vi "EndCheck Scan Code.vi"(8 "error in (no error)":errorcluster, 11 "Main":T1={"Tite"="", "Base path"=path "", "Table"=[], "Stations"=[], "Shield Array"=[], "UPHs"=[], "VISA"={"VISA"="", "baud rate"=9600, "data bits"=8, "parity"=enum."None", "stop bits"=10, "flow control"=0}, "Path"={"roof"=path "", "Config"=path "", "Png"=path ""}, "Ctr"={"DB Dispaly"=refnum, "Error Table"=refnum, "Display"=refnum, "Login"=refnum, "Exit"=refnum, "FTT_Submit"=refnum}, "Login"={"User"="", "Grade"=""}, "information"={"cause"="", "Type"=enum."Inform", "code"=0, "Suroce"="", "Status"=FALSE}, "Local DB"={"Connstr"="", "Database"={"Constr"={"Driver"="", "Server"="", "User"="", "Pwd"="", "Database"=""}, "conn ref"=refnum, "State"=FALSE}}, "Remote DB"={"Connstr"="", "Database"={"Constr"={"Driver"="", "Server"="", "User"="", "Pwd"="", "Database"=""}, "conn ref"=refnum, "State"=FALSE}}, "FTT TV"="", "ExchangeTime"=0, "NVH"="", "EOL Path"=path ""} {"VISA"."flow control" items=["None", "XON/XOFF", "RTS/CTS", "XON/XOFF & RTS/CTS", "DTR/DSR", "XON/XOFF & DTR/DSR"]; "VISA"."stop bits" items=["1.0"=10, "1.5"=15, "2.0"=20]}) -> (0 "error out":errorcluster)   [LabVIEW 2014]
uses:
  Type'def/Online_Table.ctl
  <vilib>/Instr/_visa.llb/VISA Flush IO Buffer Mask.ctl
  <vilib>/addons/database/_DB Variant To Data/Database Variant To Data.xnode
  Type'def/FTT Display Type.ctl
  Type'def/UPH Config.ctl
  VISA/Ctr/VISA Ctr.ctl
  Type'def/Main Ctr Ref.ctl
  Type'def/User Login.ctl
  Database/Ctr/Constr.ctl
  <vilib>/addons/database/Connection.llb/Conn ObjectReference.ctl
  <vilib>/addons/database/NI_Database_API.lvlib
  Database/Ctr/Conneect State.ctl
  Type'def/MainCtr.ctl
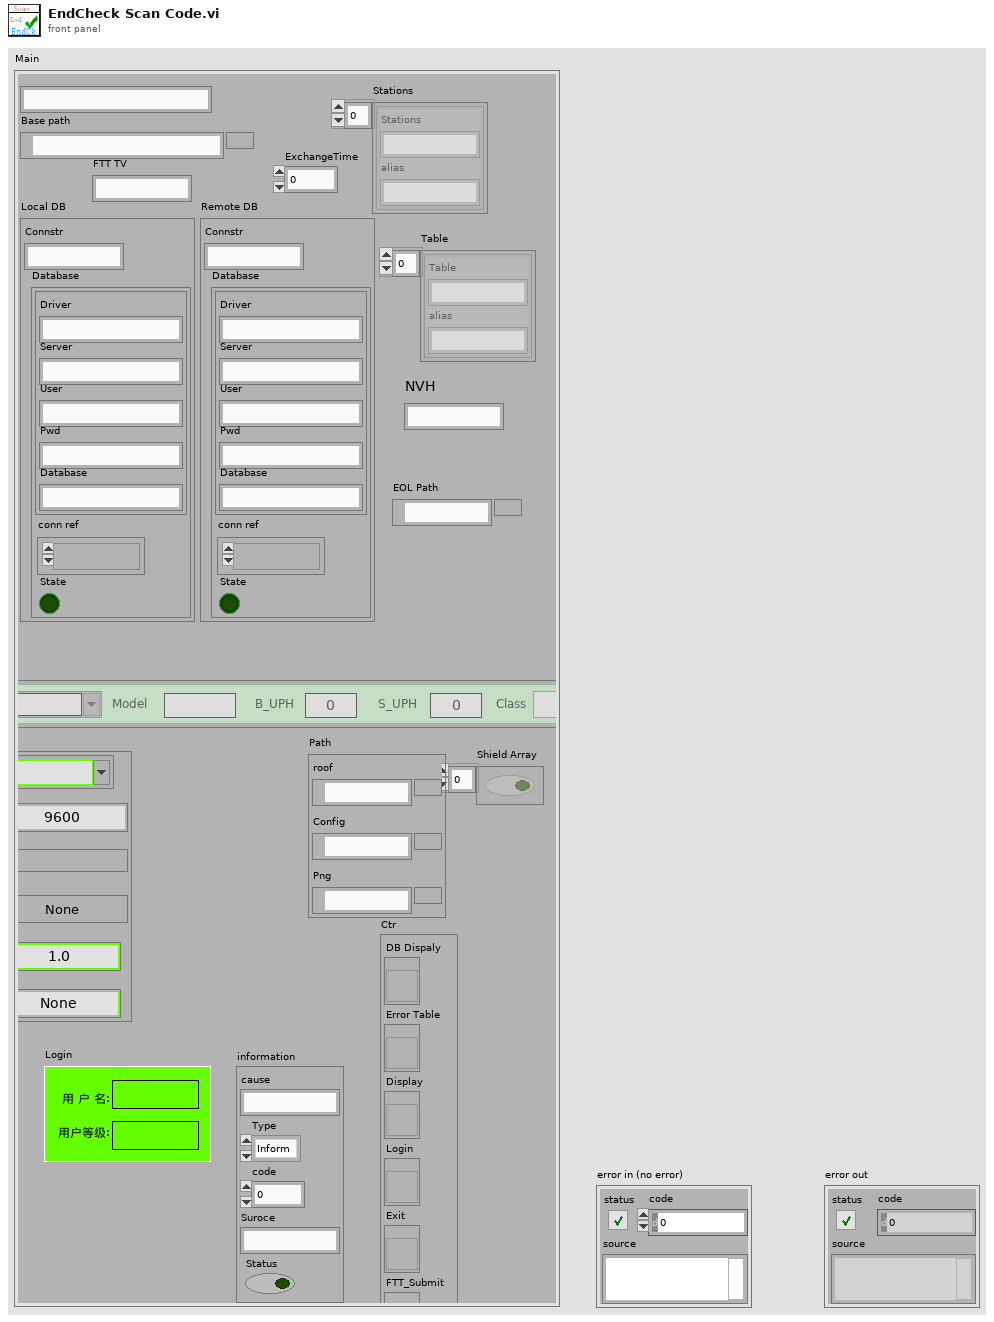
[diagram p1: front panel]
types:
  T1 = typedef "MainCtr.ctl" = cluster{"Tite":string, "Base path":path, "Table":cluster{"Table":string, "alias":string}[], "Stations":cluster{"Stations":string, "alias":string}[], "Shield Array":bool[], "UPHs":T2[], "VISA":T3, "Path":cluster{"roof":path, "Config":path, "Png":path}, "Ctr":T4, "Login":T5, "information":cluster{"cause":string, "Type":enum16{"Inform", "Warning", "Alarm"}, "code":i32, "Suroce":string, "Status":bool}, "Local DB":cluster{"Connstr":string, "Database":T6}, "Remote DB":cluster{"Connstr":string, "Database":T6}, "FTT TV":string, "ExchangeTime":i32, "NVH":string, "EOL Path":path}
  T2 = typedef "UPH Config.ctl" = cluster{"Line_No":string, "Model":string, "B_UPH ":i16, "S_UPH  ":i16, "Class":enum16{"Big", "Small"}}
  T3 = typedef "VISA Ctr.ctl" = cluster{"VISA":refnum<visa-resource-name>, "baud rate":u32, "data bits":u16, "parity":enum16{"None", "Odd", "Even", "Mark", "Space"}, "stop bits":u16, "flow control":u16}
  T4 = typedef "Main Ctr Ref.ctl" = cluster{"DB Dispaly":refnum<vi>, "Error Table":refnum<vi>, "Display":refnum<vi>, "Login":refnum<vi>, "Exit":refnum<vi>, "FTT_Submit":refnum<vi>}
  T5 = typedef "User Login.ctl" = cluster{"User":string, "Grade":string}
  T6 = typedef "Conneect State.ctl" = cluster{"Constr":T7, "conn ref":T8, "State":bool}
  T7 = typedef "Constr.ctl" = cluster{"Driver":string, "Server":string, "User":string, "Pwd":string, "Database":string}
  T8 = typedef "NI_Database_API.lvlib/Conn ObjectReference.ctl" = refnum<k1>
  T9 = typedef "FTT Display Type.ctl" = cluster{"Line.No":string, "Model":string, "Color":string, "UPH":dbl, "Plan":dbl, "Target Rate":dbl, "Target ":dbl, "Actual":dbl, "FTT":dbl, "FTT Rate":dbl, "Repaired":dbl, "Reject":dbl, "Ouline":dbl, "Line State":string}
  T10 = cluster{"cause":string, "Type":enum16{"Inform", "Warning", "Alarm"}, "code":i32, "Suroce":string, "Status":bool}
  T11 = typedef "Online_Table.ctl" = cluster{"SN":string, "Frame":string, "Station":string, "Model":string, "Color":string, "OnTime":timestamp, "OutTime":timestamp, "Repaired":i32, "OnRepair":bool, "Pstate":string}
  T12 = cluster{"Display":T9, "Main ":T1, "Online_Table":T11, "information":cluster{"cause":string, "Type":enum16{"Inform", "Warning", "Alarm"}, "code":i32, "Suroce":string, "Status":bool}}
  T13 = typedef "VISA Flush IO Buffer Mask.ctl" = u16
  T14 = cluster{"Display":T9, "Class":enum16{"Big", "Small"}}
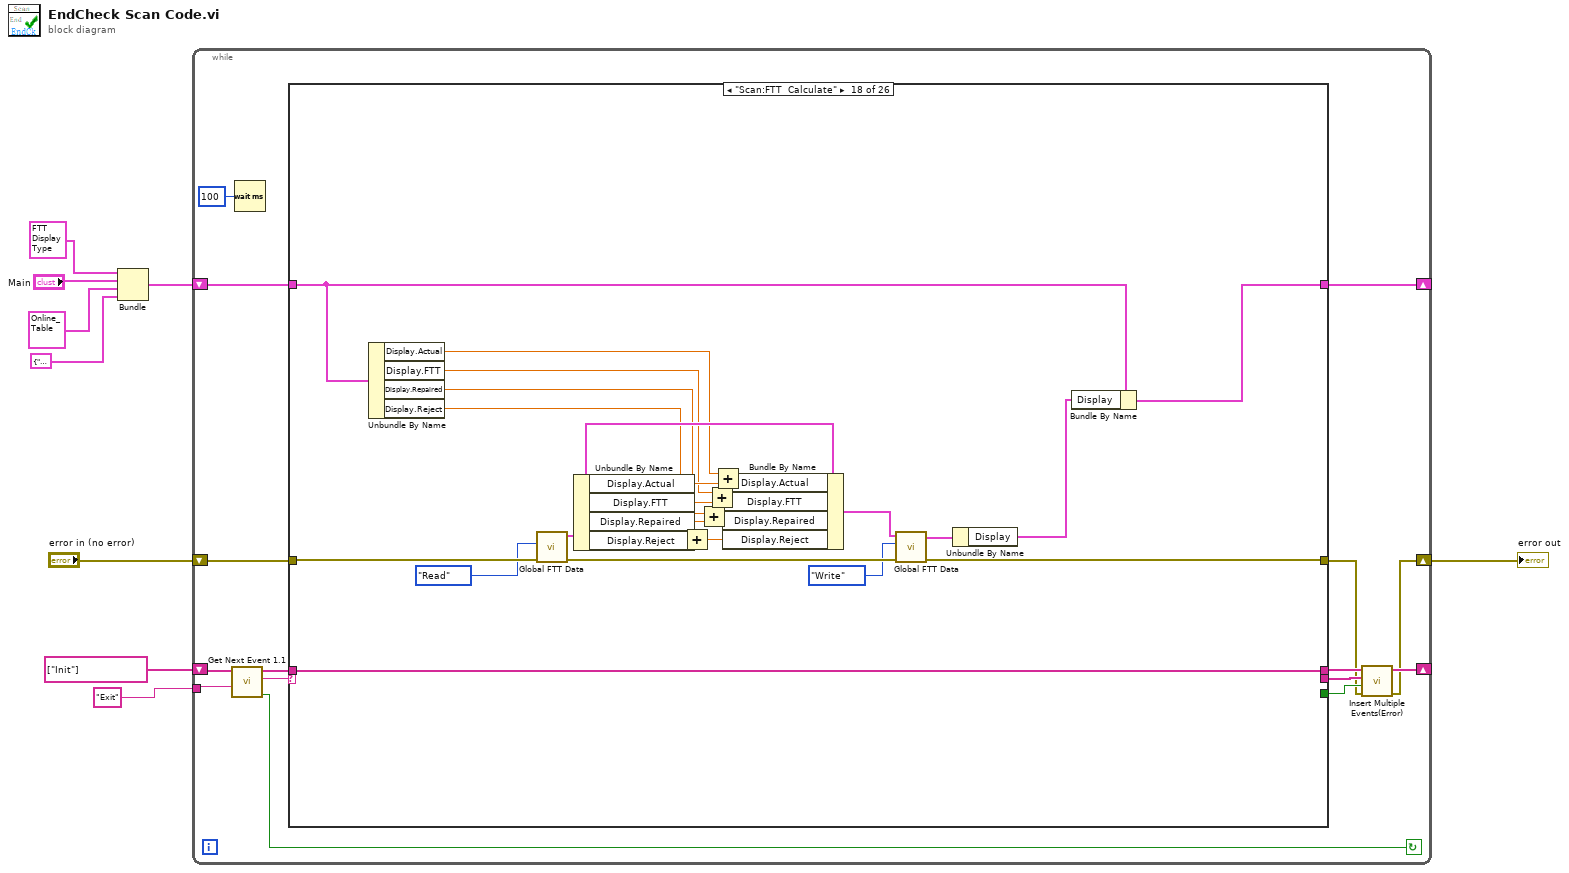
[diagram p0: block diagram]
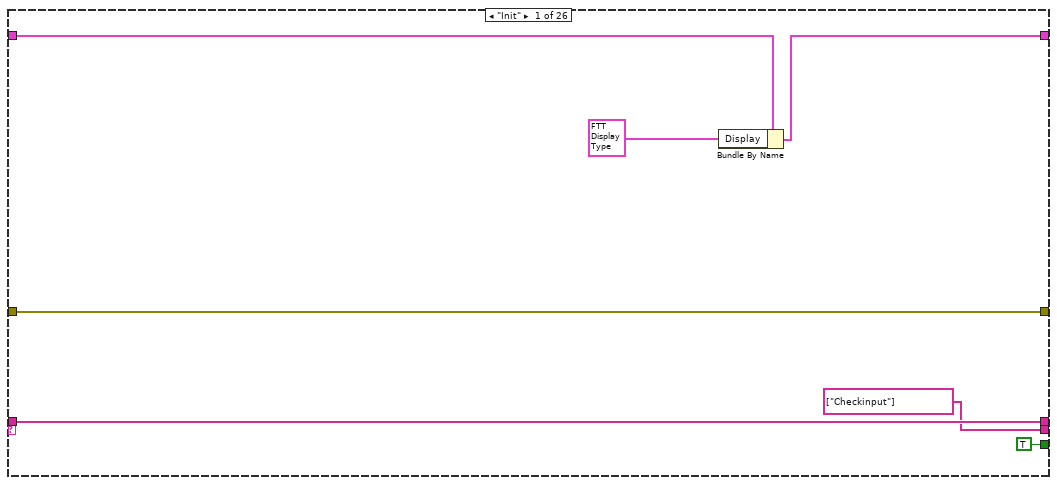
[diagram p2: hidden frame]
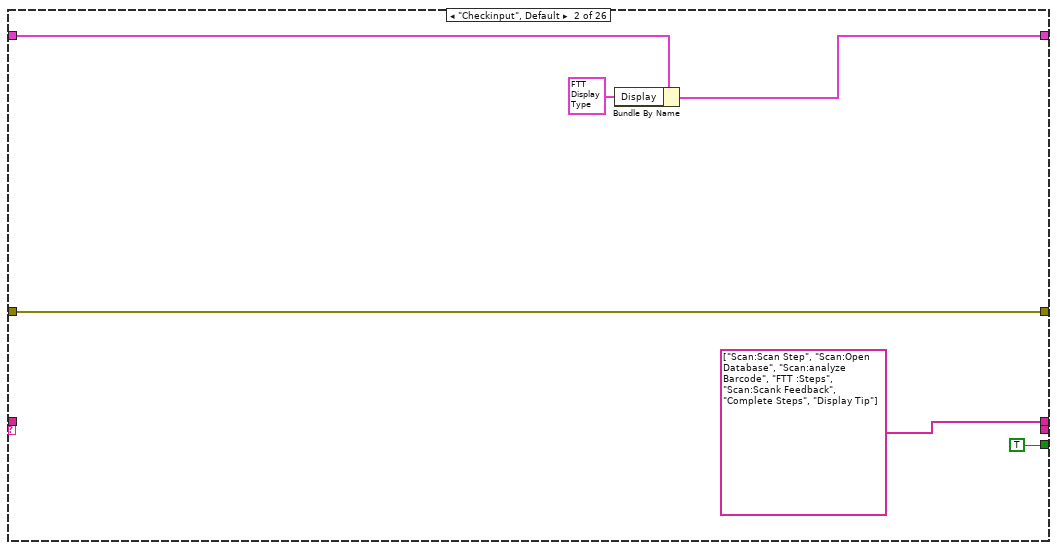
[diagram p3: hidden frame]
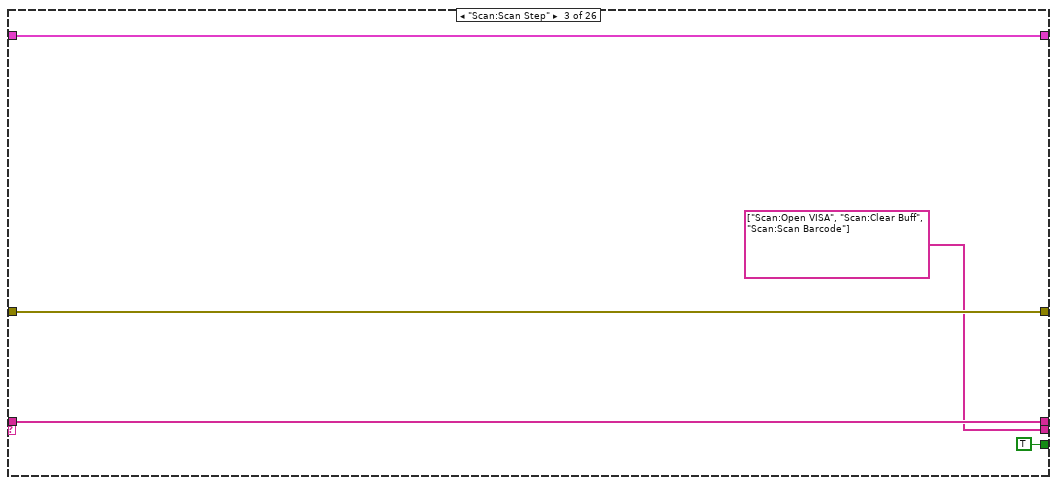
[diagram p4: hidden frame]
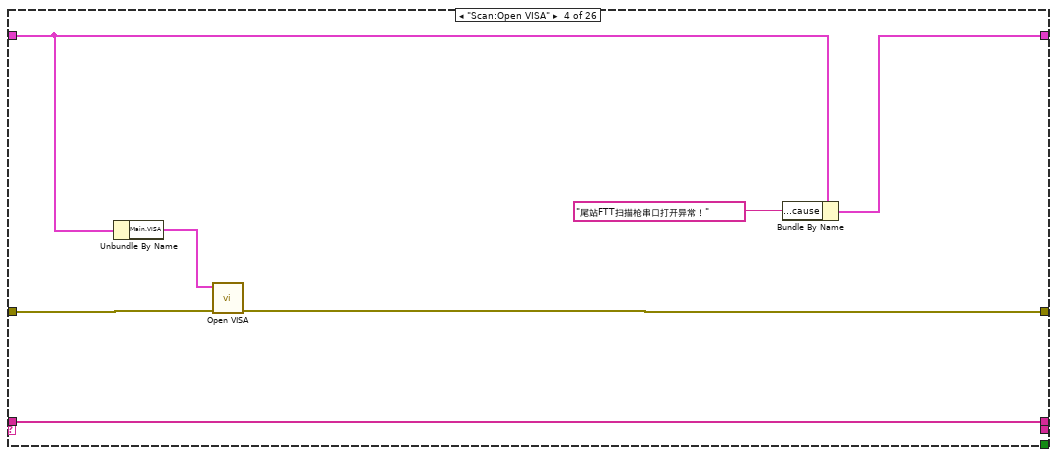
[diagram p5: hidden frame]
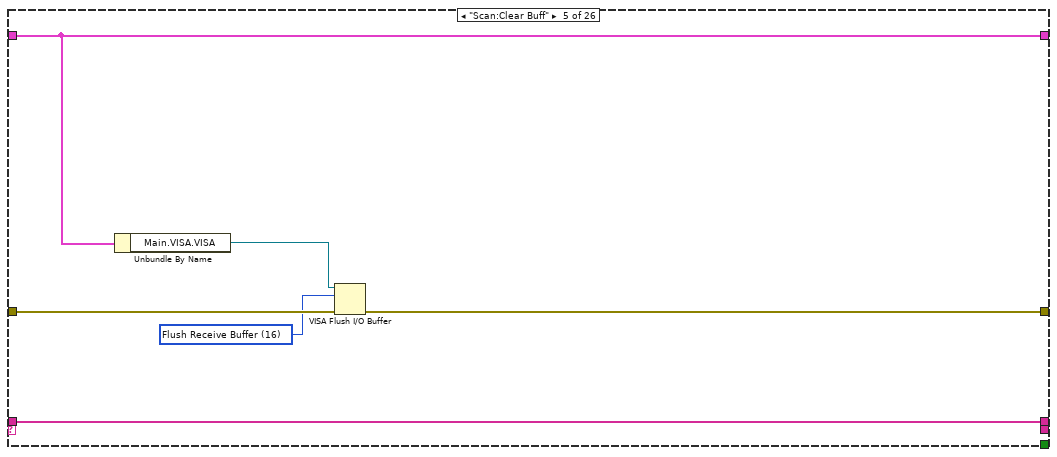
[diagram p6: hidden frame]
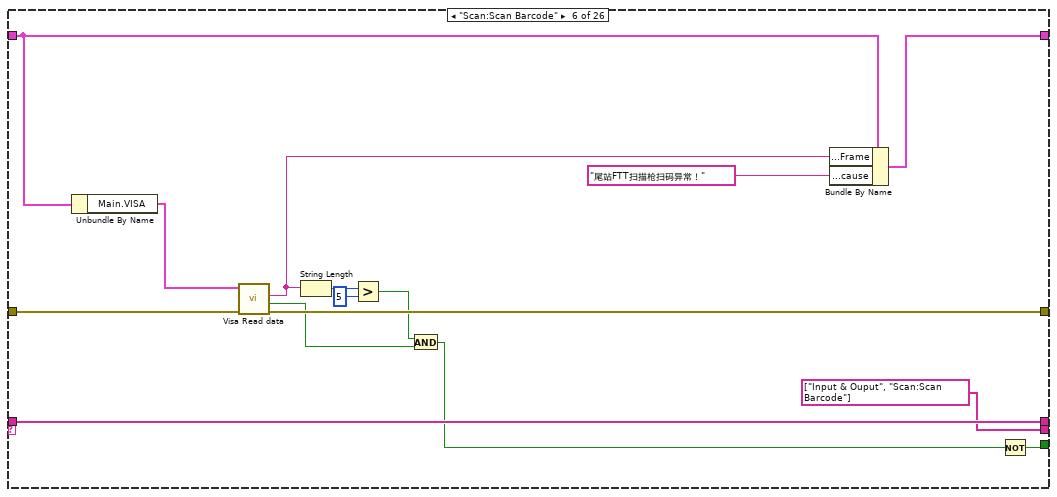
[diagram p7: hidden frame]
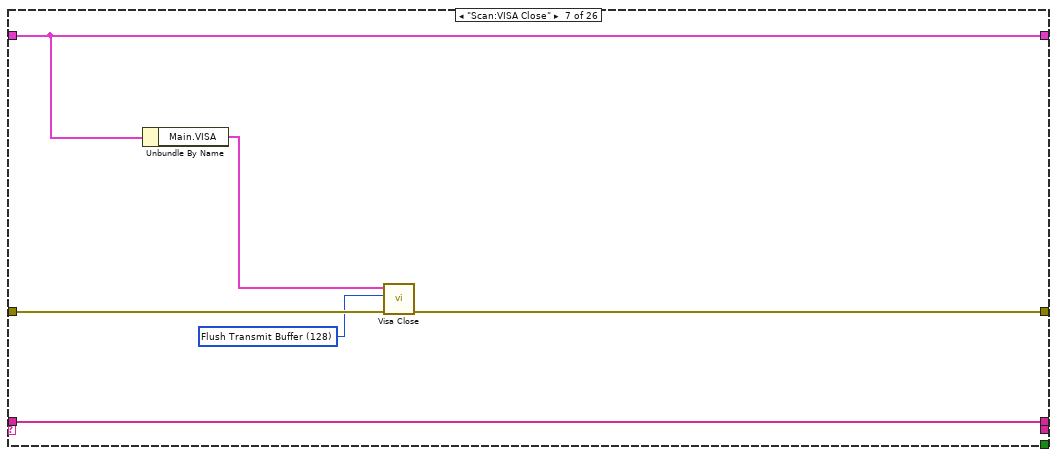
[diagram p8: hidden frame]
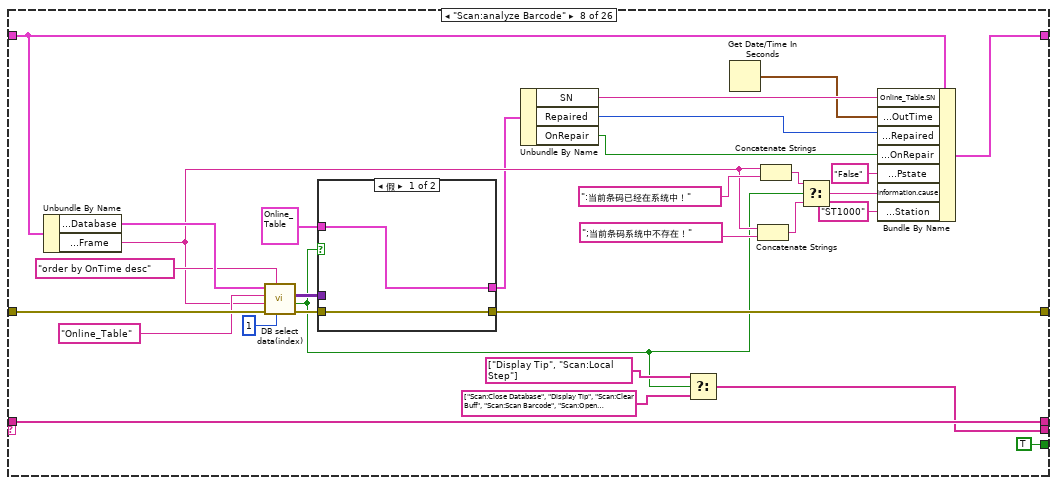
[diagram p9: hidden frame]
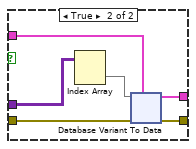
[diagram p10: hidden frame]
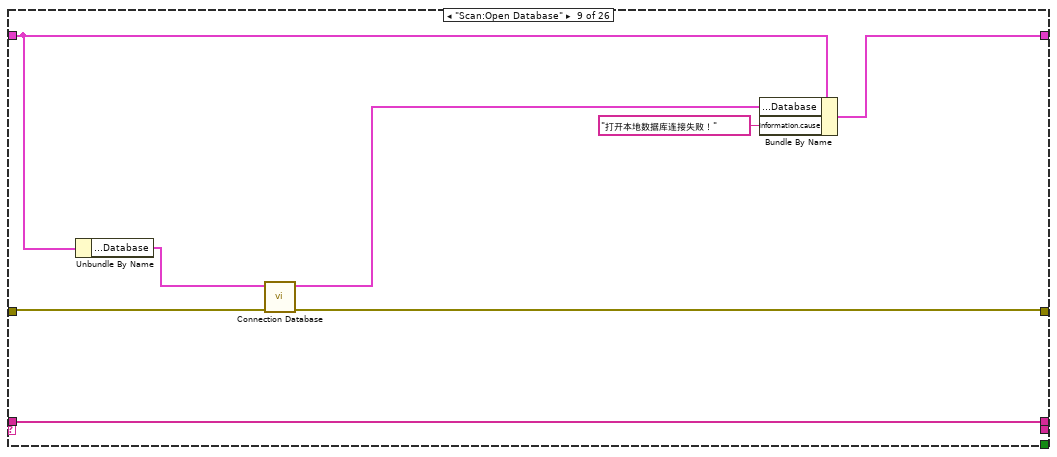
[diagram p11: hidden frame]
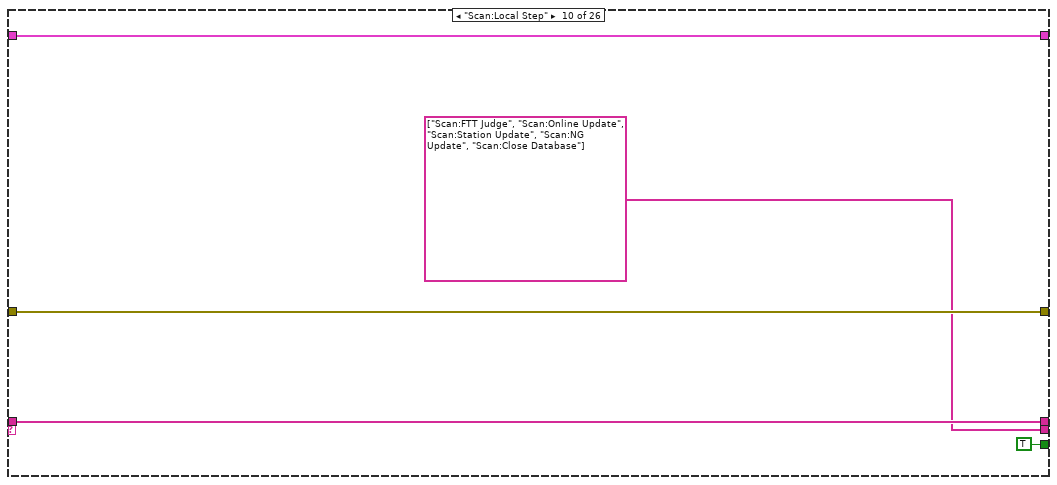
[diagram p12: hidden frame]
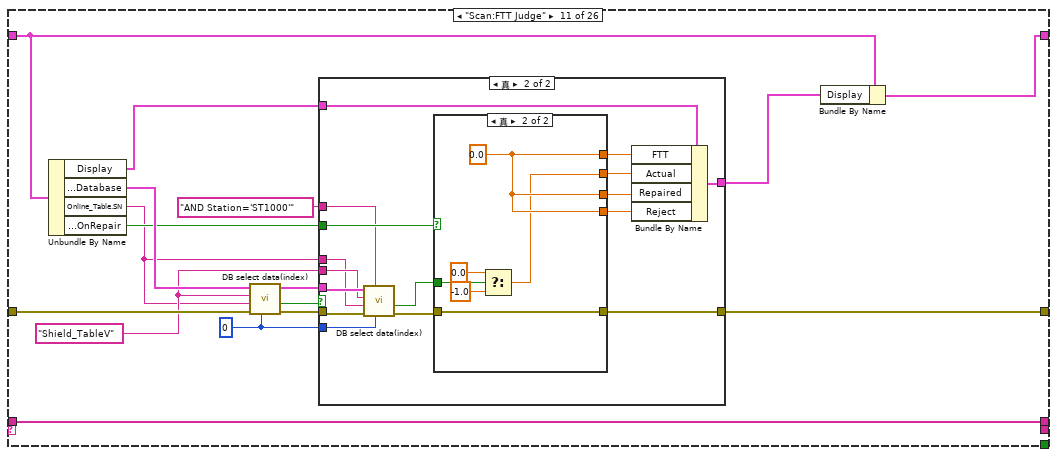
[diagram p13: hidden frame]
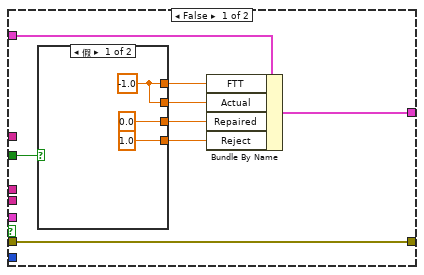
[diagram p14: hidden frame]
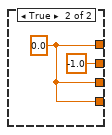
[diagram p15: hidden frame]
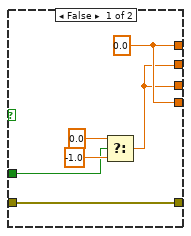
[diagram p16: hidden frame]
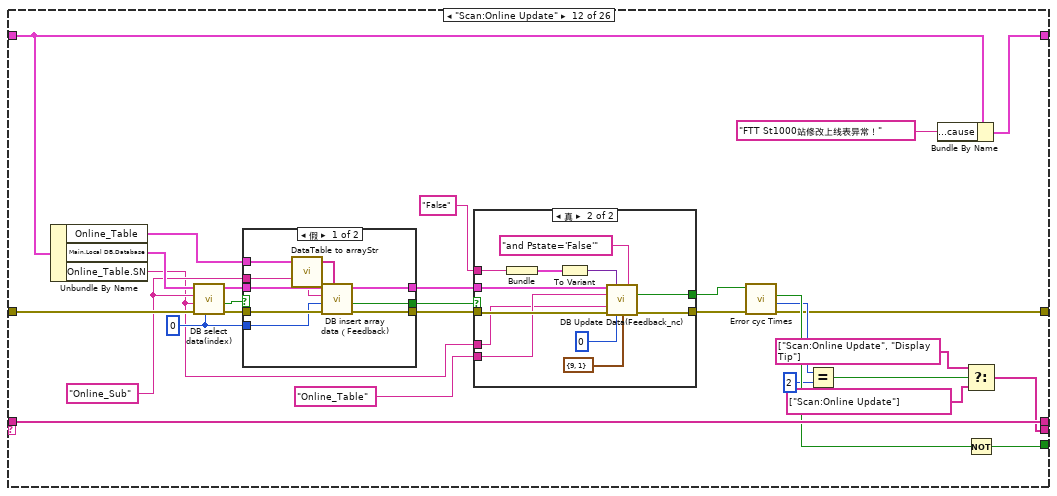
[diagram p17: hidden frame]
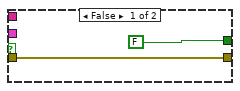
[diagram p18: hidden frame]
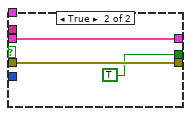
[diagram p19: hidden frame]
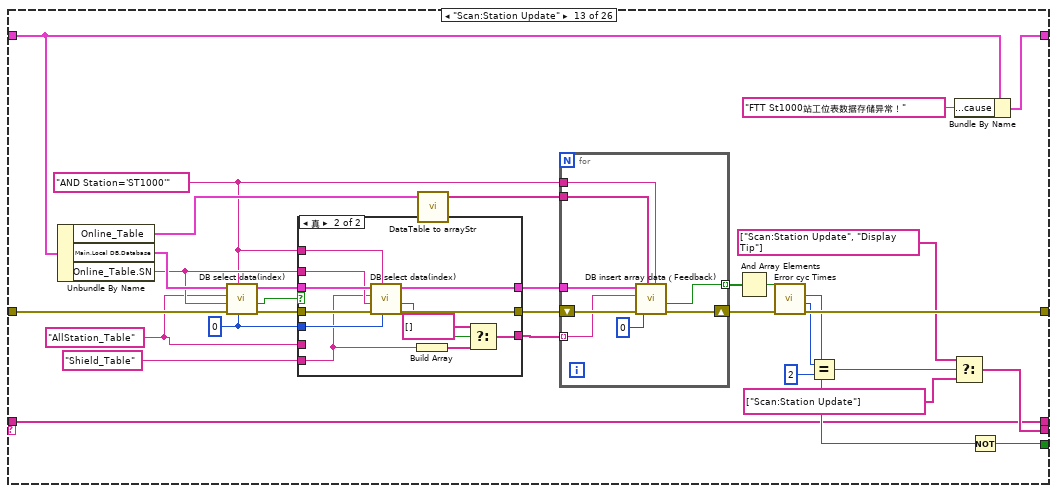
[diagram p20: hidden frame]
diagram:
  n1 = Bundle("Display"=T9 {"Line.No"="", "Model"="", "Color"="", "UPH"=0.0, "Plan"=0.0, "Target Rate"=0.0, "Target "=0.0, "Actual"=0.0, "FTT"=0.0, "FTT Rate"=0.0, "Repaired"=0.0, "Reject"=0.0, "Ouline"=0.0, "Line State"=""}, "Main"="Main", "Online_Table"=T11 {"SN"="", "Frame"="", "Station"="", "Model"="", "Color"="", "OnTime"=timestamp(0 s since 1904-01-01), "OutTime"=timestamp(0 s since 1904-01-01), "Repaired"=0, "OnRepair"=FALSE, "Pstate"=""}, "information"=T10 {"cause"="", "Type"=enum."Inform", "code"=0, "Suroce"="", "Status"=FALSE}) -> (w6:T12)  [unwired: 1 in]
  n2 = while {
    tunnel: "Exit" ("Exit Event") -> [w21]
    shift-right: [w17] -> _
    shift-left: string[] ["Init"] -> [w22]
    shift-right: [w11] -> w3
    shift-left: "error in (no error)" -> [w20]
    shift-right: [w13] -> _
    shift-left: w6 -> [w18]
    stop <- w23 continue-if-true
    n3 = call "Get Next Event 1.1.vi"("Exit Event"=w21, "event queue in"=w22) -> ("Condition (Exit:F)"=w23:bool, "next event"=w24:string, "event queue out"=w19:string[])  [unwired: 6 in, 1 out]
    n4 = Wait (ms)(milliseconds to wait=u32 100 ("等待时间（毫秒）")) -> ()  [unwired: 1 out]
    n5 = case shown="\"Scan:FTT  Calculate\"" w24 {
      tunnel: w20 -> [w30 w36 w40 w49 w54 w70 w75 w105 w462 w466 w483 w552 w610 w643 w694 w700 w706 w732 w760 w806 w811 w816 w819 w827 w832 w842]
      tunnel: w19 -> [w31 _ w41 w46 w50 w69 w72 w106 w455 w465 w481 w553 w582 w645 w695 w699 w704 w731 w761 w807 w812 w815 w821 w824 w835 _]
      tunnel: w18 -> [w29 w33 w42 w45 w55 w66 w76 w93 w459 w467 w476 w530 w593 w640 w690 w698 w702 w712 w745 w802 w813 w814 w820 w828 w837 w847]
      tunnel: [w30 w36 w40 w47 w51 w68 w74 w95 w461 w466 w473 w528 w590 w642 w692 w700 w705 w713 w739 w805 w810 w816 w819 w825 w833 w848] -> w12
      tunnel: [w31 string[] ["Scan:Scan Step", "Scan:Open Database", "Scan:analyze Barcode", "FTT :Steps", "Scan:Scank Feedback", "Complete Steps", "Display Tip"] w41 w46 w50 w69 w72 w106 w455 w465 w481 w553 w582 w645 w695 w699 w704 w731 w761 w807 w812 w815 w821 w824 w835 string[] ["Checkinput"]] -> w16
      tunnel: [TRUE ("Insert all? (T)") TRUE ("Insert all? (T)") TRUE ("Insert all? (T)") _ _ w64 _ TRUE ("Insert all? (T)") _ TRUE ("Insert all? (T)") _ w538 w594 w644 _ TRUE ("Insert all? (T)") _ _ w753 _ _ _ TRUE ("Insert all? (T)") w823 FALSE ("Insert all? (T)") TRUE ("Insert all? (T)")] -> w15
      tunnel: [string[] ["Checkinput"] _ string[] ["Scan:Open VISA", "Scan:Clear Buff", "Scan:Scan Barcode"] _ _ string[] ["Input & Ouput", "Scan:Scan Barcode"] _ w97 _ string[] ["Scan:FTT Judge", "Scan:Online Update", "Scan:Station Update", "Scan:NG Update", "Scan:Close Database"] _ w531 w584 w641 _ string[] ["FTT :Open database", "Scan:FTT  Calculate", "FTT:Data Save", "FTT:Close database"] _ _ w750 _ _ _ string[] ["Scan:VISA Close", "Exit"] string[] ["Quit"] _ string[] ["Scan:Close Database", "FTT:Close database", "Scan:VISA Close"]] -> w14
      tunnel: [w28 w32 w42 w44 w55 w65 w76 w92 w458 w467 w475 w529 w592 w639 w689 w698 w703 w711 w744 w801 w813 w814 w820 w828 w837 w847] -> w13
      frame "Init" {
        n6 = Bundle By Name(cluster=w29, "Display"=T9 {"Line.No"="", "Model"="", "Color"="", "UPH"=0.0, "Plan"=0.0, "Target Rate"=0.0, "Target "=0.0, "Actual"=0.0, "FTT"=0.0, "FTT Rate"=0.0, "Repaired"=0.0, "Reject"=0.0, "Ouline"=0.0, "Line State"=""}) -> (w28:T12)
      }
      frame "Checkinput", Default {
        n7 = Bundle By Name(cluster=w33, "Display"=T9 {"Line.No"="", "Model"="", "Color"="", "UPH"=0.0, "Plan"=0.0, "Target Rate"=0.0, "Target "=0.0, "Actual"=0.0, "FTT"=0.0, "FTT Rate"=0.0, "Repaired"=0.0, "Reject"=0.0, "Ouline"=0.0, "Line State"=""}) -> (w32:T12)
      }
      frame "Scan:Scan Step" {
      }
      frame "Scan:Open VISA" {
        n8 = Unbundle By Name(w45) -> ("Main.VISA"=w48:T3)
        n9 = call "Open VISA.vi"("错误输入（无错误）"=w49, "VISA"=w48) -> ("error out"=w47:errorcluster)  [unwired: 8 in, 1 out]
        n10 = Bundle By Name(cluster=w45, "Main.information.cause"="尾站FTT扫描枪串口打开异常！" ("Main .information.cause")) -> (w44:T12)
      }
      frame "Scan:Clear Buff" {
        w52 = T13 16 items=["Flush Receive Buffer"=16, "Write Transmit Buffer to Device"=32, "Flush Receive Buffer (No I/O)"=64, "Flush Transmit Buffer"=128] ("Mask")
        n11 = Unbundle By Name(w55) -> ("Main.VISA.VISA"=w53:refnum<visa-resource-name>)
        n12 = VISA Flush I/O Buffer(VISA resource name=w53, mask (16)=w52, error in (no error)=w54) -> (error out=w51:errorcluster)  [unwired: 1 out]
      }
      frame "Scan:Scan Barcode" {
        n13 = Unbundle By Name(w66) -> ("Main.VISA"=w67:T3)
        n14 = call "Visa Read data.vi"("错误输入（无错误）"=w70, "VISA Name"=w67) -> ("error out"=w68:errorcluster, "State"=w57:bool, "trimmed string"=w61:string)  [unwired: 6 in, 1 out]
        n15 = String Length(string=w61) -> (length=w60:i32)
        n16 = Greater?(x=w60, y=5) -> (0:w58:bool)
        n17 = And(x=w58, y=w57) -> (x .and. y?=w56:bool)
        n18 = Bundle By Name(cluster=w66, "Online_Table.Frame"=w61, "information.cause"="尾站FTT扫描枪扫码异常！") -> (w65:T12)
        n19 = Not(x=w56) -> (.not. x?=w64:bool)
      }
      frame "Scan:VISA Close" {
        w71 = T13 128 items=["Flush Receive Buffer"=16, "Write Transmit Buffer to Device"=32, "Flush Receive Buffer (No I/O)"=64, "Flush Transmit Buffer"=128] ("Mask")
        n20 = Unbundle By Name(w76) -> ("Main.VISA"=w73:T3)
        n21 = call "Visa Close.vi"("错误输入（无错误）"=w75, "Mask"=w71, "VISA"=w73) -> ("错误输出"=w74:errorcluster)  [unwired: 8 in]
      }
      frame "Scan:analyze Barcode" {
        n22 = Unbundle By Name(w93) -> ("Main.Local DB.Database"=w104:T6, "Online_Table.Frame"=w86:string)
        n23 = call "DB select data(index).vi"("index"=1, "Condtion"="order by OnTime desc", "error in (no error)"=w105, "Code"=w86, "Tabe"="Online_Table", "Connncet State"=w104) -> ("error out"=w96:errorcluster, "state"=w78:bool, "data"=w94:variant[][])  [unwired: 2 in, 1 out]
        n24 = case shown="假" w78 {
          tunnel: w96 -> [w108 w114]
          tunnel: [w108 w113] -> w95
          tunnel: w94 -> [_ w112]
          tunnel: [w107 w110] -> w80
          tunnel: T11 {"SN"="", "Frame"="", "Station"="", "Model"="", "Color"="", "OnTime"=timestamp(0 s since 1904-01-01), "OutTime"=timestamp(0 s since 1904-01-01), "Repaired"=0, "OnRepair"=FALSE, "Pstate"=""} ("Online_Table") -> [w107 w109]
          frame False {
          }
          frame True {
            n25 = Index Array(array=w112) -> (element=w111:variant[])  [unwired: 2 in]
            n26 = xnode "Database Variant To Data"("database variant"=w111, "error in (no error)"=w114, "type"=w109) -> ("data"=w110:T11, "error out"=w113:errorcluster)
          }
        }
        n27 = Unbundle By Name(w80) -> ("SN"=w85:string, "Repaired"=w84:i32, "OnRepair"=w83:bool)
        n28 = Select(t=string[] ["Display Tip", "Scan:Local Step"], s=w78, f=string[] ["Scan:Close Database", "Display Tip", "Scan:Clear Buff", "Scan:Scan Barcode", "Scan:Open Database", "Scan:analyze Barcode"]) -> (s? t:f=w97:string[])
        n29 = Get Date/Time In Seconds() -> (seconds since 1Jan1904=w81:timestamp)
        n30 = Concatenate Strings(w86, ";当前条码系统中不存在！") -> (w89:string)
        n31 = Concatenate Strings(w86, ":当前条码已经在系统中！") -> (w87:string)
        n32 = Select(t=w87, s=w78, f=w89) -> (s? t:f=w91:string)
        n33 = Bundle By Name(cluster=w93, "Online_Table.SN"=w85, "Online_Table.OutTime"=w81, "Online_Table.Repaired"=w84, "Online_Table.OnRepair"=w83, "Online_Table.Pstate"="False", "information.cause"=w91, "Online_Table.Station"="ST1000") -> (w92:T12)
      }
      frame "Scan:Open Database" {
        n34 = Unbundle By Name(w459) -> ("Main.Local DB.Database"=w460:T6)
        n35 = call "Connection Database.vi"("error in (no error)"=w462, "Connncet State"=w460) -> ("error out"=w461:errorcluster, "Connncet State out"=w457:T6)  [unwired: 8 in]
        n36 = Bundle By Name(cluster=w459, "Main.Local DB.Database"=w457, "information.cause"="打开本地数据库连接失败！") -> (w458:T12)
      }
      frame "Scan:Local Step" {
      }
      frame "Scan:FTT Judge" {
        w468 = 0 ("index")
        w471 = "Shield_TableV"
        n37 = Unbundle By Name(w476) -> ("Display"=w477:T9, "Main.Local DB.Database"=w482:T6, "Online_Table.SN"=w470:string, "Online_Table.OnRepair"=w478:bool)
        n38 = call "DB select data(index).vi"("index"=w468, "error in (no error)"=w483, "Code"=w470, "Tabe"=w471, "Connncet State"=w482) -> ("error out"=w479:errorcluster, "state"=w480:bool, "Connncet State out"=w472:T6)  [unwired: 3 in, 1 out]
        n39 = case shown="真" w480 {
          tunnel: w479 -> [w489 w504]
          tunnel: w478 -> [w490 w510]
          tunnel: w477 -> [w491 w512]
          tunnel: [w489 w505] -> w473
          tunnel: [w484 w511] -> w474
          tunnel: w472 -> [_ w502]
          tunnel: w471 -> [_ w500]
          tunnel: w470 -> [_ w499]
          tunnel: "AND Station='ST1000'" -> [_ w501]
          tunnel: w468 -> [_ w498]
          frame False {
            n40 = case shown="假" w490 {
              tunnel: [w494 w496] -> w488
              tunnel: [w494 -1.0] -> w487
              tunnel: [1.0 w496] -> w486
              tunnel: [0.0 w496] -> w485
              frame False {
                w494 = -1.0
              }
              frame True {
                w496 = 0.0
              }
            }
            n41 = Bundle By Name(cluster=w491, "FTT"=w488, "Actual"=w487, "Repaired"=w485, "Reject"=w486) -> (w484:T9)
          }
          frame True {
            n42 = call "DB select data(index).vi"("index"=w498, "Condtion"=w501, "error in (no error)"=w504, "Code"=w499, "Tabe"=w500, "Connncet State"=w502) -> ("error out"=w503:errorcluster, "state"=w497:bool)  [unwired: 2 in, 2 out]
            n43 = case shown="真" w510 {
              tunnel: [w516 w523] -> w509
              tunnel: [w515 w523] -> w508
              tunnel: [w516 w523] -> w507
              tunnel: [w515 w521] -> w506
              tunnel: w503 -> [w514 w524]
              tunnel: [w514 w524] -> w505
              tunnel: w497 -> [w513 w522]
              frame False {
                w516 = 0.0
                n44 = Select(t=0.0, s=w513, f=-1.0) -> (s? t:f=w515:dbl)
              }
              frame True {
                w523 = 0.0
                n45 = Select(t=0.0, s=w522, f=-1.0) -> (s? t:f=w521:dbl)
              }
            }
            n46 = Bundle By Name(cluster=w512, "FTT"=w509, "Actual"=w506, "Repaired"=w508, "Reject"=w507) -> (w511:T9)
          }
        }
        n47 = Bundle By Name(cluster=w476, "Display"=w474) -> (w475:T12)
      }
      frame "Scan:Online Update" {
        w547 = 0 ("index")
        w543 = "Online_Sub"
        n48 = Unbundle By Name(w530) -> ("Online_Table"=w541:T11, "Main.Local DB.Database"=w551:T6, "Online_Table.SN"=w542:string)
        n49 = call "DB select data(index).vi"("index"=w547, "error in (no error)"=w552, "Code"=w542, "Tabe"=w543, "Connncet State"=w551) -> ("error out"=w550:errorcluster, "state"=w549:bool, "Connncet State out"=w548:T6)  [unwired: 3 in, 1 out]
        n50 = case shown="假" w549 {
          tunnel: w550 -> [w576 w578]
          tunnel: w548 -> [w575 w579]
          tunnel: w543 -> [w574 _]
          tunnel: w547 -> [w573 _]
          tunnel: w541 -> [w572 _]
          tunnel: [w570 TRUE] -> w545
          tunnel: [w569 w578] -> w546
          tunnel: [w568 w579] -> w544
          frame False {
            n51 = call "DataTable to arrayStr.vi"("Online_Table"=w572) -> ("appended array"=w571:string[])  [unwired: 4 in]
            n52 = call "DB insert array data（Feedback).vi"("Data"=w571, "error in (no error)"=w576, "index"=w573, "table"=w574, "Connncet State"=w575) -> ("error out"=w569:errorcluster, "state"=w570:bool, "Connncet State out"=w568:T6)  [unwired: 4 in]
          }
          frame True {
          }
        }
        n53 = case shown="真" w545 {
          tunnel: w546 -> [w555 w567]
          tunnel: w544 -> [_ w565]
          tunnel: [w555 w566] -> w540
          tunnel: "Online_Table" -> [_ w564]
          tunnel: w542 -> [_ w563]
          tunnel: [FALSE w560] -> w539
          tunnel: "False" -> [_ w559]
          frame False {
          }
          frame True {
            n54 = Bundle(w559) -> (w558:cluster{string})  [unwired: 1 in]
            n55 = To Variant(anything=w558) -> (Variant=w557:variant)
            n56 = call "DB Update Data(Feedback_nc).vi"("Connncet State"=w565, "data"=w557, "Sel"="and Pstate='False'", "table"=w564, "Code"=w563, "error in (no error)"=w567, "Sel index"=0, "Pos"=cluster{"index":i32, "Len":i32} {"index"=9, "Len"=1}) -> ("State"=w560:bool, "error out"=w566:errorcluster)  [unwired: 5 in, 1 out]
          }
        }
        n57 = call "Error cyc Times.vi"("error in (no error)"=w540, "Status in"=w539) -> ("error out"=w528:errorcluster, "Numeric"=w536:i32, "Cys Status"=w537:bool)  [unwired: 6 in, 1 out]
        n58 = Equal?(x=w536, y=2) -> (x = y?=w534:bool)
        n59 = Bundle By Name(cluster=w530, "information.cause"="FTT St1000站修改上线表异常！") -> (w529:T12)
        n60 = Select(t=string[] ["Scan:Online Update", "Display Tip"], s=w534, f=string[] ["Scan:Online Update"]) -> (s? t:f=w531:string[])
        n61 = Not(x=w537) -> (.not. x?=w538:bool)
      }
      frame "Scan:Station Update" {
        w603 = 0 ("index")
        w596 = "AND Station='ST1000'"
        w602 = "AllStation_Table"
        n62 = Unbundle By Name(w593) -> ("Online_Table"=w598:T11, "Main.Local DB.Database"=w609:T6, "Online_Table.SN"=w604:string)
        n63 = call "DB select data(index).vi"("index"=w603, "Condtion"=w596, "error in (no error)"=w610, "Code"=w604, "Tabe"=w602, "Connncet State"=w609) -> ("error out"=w608:errorcluster, "state"=w607:bool, "Connncet State out"=w606:T6)  [unwired: 2 in, 1 out]
        n64 = case shown="真" w607 {
          tunnel: w608 -> [w623 w635]
          tunnel: w606 -> [w619 w634]
          tunnel: "Shield_Table" -> [w621 w627]
          tunnel: w604 -> [_ w633]
          tunnel: w596 -> [_ w632]
          tunnel: w603 -> [_ w631]
          tunnel: w602 -> [w622 _]
          tunnel: [w623 w630] -> w601
          tunnel: [w620 w626] -> w599
          tunnel: [w619 w624] -> w600
          frame False {
            n65 = Build Array(w622, w621) -> (w620:string[])
          }
          frame True {
            n66 = call "DB select data(index).vi"("index"=w631, "Condtion"=w632, "error in (no error)"=w635, "Code"=w633, "Tabe"=w627, "Connncet State"=w634) -> ("error out"=w630:errorcluster, "state"=w629:bool, "Connncet State out"=w624:T6)  [unwired: 2 in, 1 out]
            n67 = Build Array(w627) -> (w628:string[])
            n68 = Select(t=string[] [], s=w629, f=w628) -> (s? t:f=w626:string[])
          }
        }
        n69 = call "DataTable to arrayStr.vi"("Online_Table"=w598) -> ("appended array"=w597:string[])  [unwired: 4 in]
        n70 = for {
          tunnel: w600 -> [w617]
          tunnel: w599 -> [w616] mode=indexing
          tunnel: w597 -> [w615]
          tunnel: w596 -> [w613]
          shift-right: [w612] -> w591
          shift-left: w601 -> [w618]
          tunnel: [w611] -> w595 mode=indexing
          n71 = call "DB insert array data（Feedback).vi"("Condtion"=w613, "Data"=w615, "error in (no error)"=w618, "index"=0, "table"=w616, "Connncet State"=w617) -> ("error out"=w612:errorcluster, "state"=w611:bool)  [unwired: 3 in, 1 out]
        }
        n72 = And Array Elements(Boolean array=w595) -> (logical AND=w589:bool)
        n73 = call "Error cyc Times.vi"("error in (no error)"=w591, "Status in"=w589) -> ("error out"=w590:errorcluster, "Numeric"=w587:i32, "Cys Status"=w588:bool)  [unwired: 6 in, 1 out]
        n74 = Equal?(x=w587, y=2) -> (x = y?=w585:bool)
        n75 = Select(t=string[] ["Scan:Station Update", "Display Tip"], s=w585, f=string[] ["Scan:Station Update"]) -> (s? t:f=w584:string[])
        n76 = Bundle By Name(cluster=w593, "information.cause"="FTT St1000站工位表数据存储异常！") -> (w592:T12)
        n77 = Not(x=w588) -> (.not. x?=w594:bool)
      }
      frame "Scan:NG Update" {
        w660 = 0 ("index")
        w637 = "NG_Table"
        n78 = Unbundle By Name(w640) -> ("Online_Table"=w656:T11, "Main.Local DB.Database"=w665:T6, "Online_Table.SN"=w661:string)
        n79 = call "DB select data(index).vi"("index"=w660, "error in (no error)"=w643, "Code"=w661, "Tabe"=w637, "Connncet State"=w665) -> ("error out"=w664:errorcluster, "state"=w663:bool, "Connncet State out"=w662:T6)  [unwired: 3 in, 1 out]
        n80 = case shown="真" w663 {
          tunnel: w664 -> [w677 w688]
          tunnel: w662 -> [w673 w687]
          tunnel: "NG_Shield" -> [w675 w681]
          tunnel: w661 -> [_ w686]
          tunnel: w660 -> [_ w685]
          tunnel: w637 -> [w676 _]
          tunnel: [w677 w684] -> w659
          tunnel: [w674 w680] -> w657
          tunnel: [w673 w678] -> w658
          frame False {
            n81 = Build Array(w676, w675) -> (w674:string[])
          }
          frame True {
            n82 = call "DB select data(index).vi"("index"=w685, "error in (no error)"=w688, "Code"=w686, "Tabe"=w681, "Connncet State"=w687) -> ("error out"=w684:errorcluster, "state"=w683:bool, "Connncet State out"=w678:T6)  [unwired: 3 in, 1 out]
            n83 = Build Array(w681) -> (w682:string[])
            n84 = Select(t=string[] [], s=w683, f=w682) -> (s? t:f=w680:string[])
          }
        }
        n85 = call "DataTable to arrayStr.vi"("Online_Table"=w656) -> ("appended array"=w655:string[])  [unwired: 4 in]
        n86 = for {
          tunnel: w658 -> [w671]
          tunnel: w657 -> [w670] mode=indexing
          tunnel: w655 -> [w669]
          shift-right: [w667] -> w653
          shift-left: w659 -> [w672]
          tunnel: [w666] -> w654 mode=indexing
          n87 = call "DB insert array data（Feedback).vi"("Data"=w669, "error in (no error)"=w672, "index"=0, "table"=w670, "Connncet State"=w671) -> ("error out"=w667:errorcluster, "state"=w666:bool)  [unwired: 4 in, 1 out]
        }
        n88 = And Array Elements(Boolean array=w654) -> (logical AND=w652:bool)
        n89 = call "Error cyc Times.vi"("error in (no error)"=w653, "Status in"=w652) -> ("error out"=w642:errorcluster, "Numeric"=w650:i32, "Cys Status"=w651:bool)  [unwired: 6 in, 1 out]
        n90 = Equal?(x=w650, y=2) -> (x = y?=w648:bool)
        n91 = Bundle By Name(cluster=w640, "information.cause"="FTT St1000站NG表数据存储异常！") -> (w639:T12)
        n92 = Select(t=string[] ["Scan:NG Update", "Display Tip"], s=w648, f=string[] ["Scan:NG Update"]) -> (s? t:f=w641:string[])
        n93 = Not(x=w651) -> (.not. x?=w644:bool)
      }
      frame "Scan:Close Database" {
        n94 = Unbundle By Name(w690) -> ("Main.Local DB.Database"=w693:T6)
        n95 = call "Disconncetion DB.vi"("error in (no error)"=w694, "Connncet State"=w693) -> ("error out"=w692:errorcluster, "Connect State"=w691:T6)  [unwired: 8 in]
        n96 = Bundle By Name(cluster=w690, "Main.Local DB.Database"=w691) -> (w689:T12)
      }
      frame "FTT :Steps" {
      }
      frame "FTT :Open database" {
        n97 = Unbundle By Name(w702) -> ("Main.Local DB.Database"=w701:T6)
        n98 = call "Connection Database.vi"("error in (no error)"=w706, "Connncet State"=w701) -> ("error out"=w705:errorcluster, "Connncet State out"=w708:T6)  [unwired: 8 in]
        n99 = Bundle By Name(cluster=w702, "Main.Local DB.Database"=w708, "information.cause"="打开远程数据库连接失败！") -> (w703:T12)
      }
      frame "Scan:FTT  Calculate" {
        n100 = Unbundle By Name(w712) -> ("Display.Actual"=w726:dbl, "Display.FTT"=w723:dbl, "Display.Repaired"=w720:dbl, "Display.Reject"=w717:dbl)
        n101 = call "Global FTT Data.vi"("error in (no error)"=w732, "Mode"=enum16{"Read", "Write"}."Read") -> ("error out"=w716:errorcluster, "Cluster"=w727:T14)  [unwired: 8 in]
        n102 = Unbundle By Name(w727) -> ("Display.Actual"=w728:dbl, "Display.FTT"=w724:dbl, "Display.Repaired"=w721:dbl, "Display.Reject"=w718:dbl)
        n103 = Add(x=w717, y=w718) -> (x+y=w719:dbl)
        n104 = Add(x=w720, y=w721) -> (x+y=w722:dbl)
        n105 = Add(x=w723, y=w724) -> (x+y=w725:dbl)
        n106 = Add(x=w726, y=w728) -> (x+y=w729:dbl)
        n107 = Bundle By Name(cluster=w727, "Display.Actual"=w729, "Display.FTT"=w725, "Display.Repaired"=w722, "Display.Reject"=w719) -> (w715:T14)
        n108 = call "Global FTT Data.vi"("error in (no error)"=w716, "Mode"=enum16{"Read", "Write"}."Write", "Display"=w715) -> ("error out"=w713:errorcluster, "Cluster"=w710:T14)  [unwired: 7 in]
        n109 = Unbundle By Name(w710) -> ("Display"=w709:T9)
        n110 = Bundle By Name(cluster=w712, "Display"=w709) -> (w711:T12)
      }
      frame "FTT:Data Save" {
        n111 = Unbundle By Name(w745) -> ("Online_Table.SN"=w740:string, "Online_Table.Station"=w742:string, "Display"=w741:T9, "Main.Local DB.Database"=w757:T6, "Display.Line.No"=w756:string)
        n112 = First Call?() -> (First Call?: T/F=w759:bool)
        n113 = case shown="假" w759 {
          tunnel: w760 -> [w770 w782]
          tunnel: "[FTT_Clinet].[dbo].[FTT1_ Write]" -> [w768 w777]
          tunnel: w757 -> [w769 w781]
          tunnel: w756 -> [w767 w774]
          tunnel: w741 -> [w766 w773]
          tunnel: [w763 w775] -> w755
          tunnel: [w762 w772] -> w754
          frame False {
            n114 = call "DB Update Data(Feedback).vi"("Pos"=cluster{"index":i32, "Len":i32} {"index"=0, "Len"=14}, "Sel index"=0, "data"=w766, "error in (no error)"=w770, "Code"=w767, "table"=w768, "Connncet State"=w769) -> ("error out"=w763:errorcluster, "State"=w762:bool)  [unwired: 2 in, 1 out]
          }
          frame True {
            n115 = call "ftt array.vi"("Display"=w773) -> ("appended array"=w776:string[])  [unwired: 4 in]
            n116 = call "DB select data(index).vi"("index"=0, "error in (no error)"=w782, "Code"=w774, "Tabe"=w777, "Connncet State"=w781) -> ("error out"=w780:errorcluster, "state"=w779:bool, "Connncet State out"=w778:T6)  [unwired: 3 in, 1 out]
            n117 = case shown="假" w779 {
              tunnel: w780 -> [w790 w799]
              tunnel: w778 -> [w789 w798]
              tunnel: w777 -> [w788 w797]
              tunnel: w776 -> [w786 _]
              tunnel: [w785 w793] -> w775
              tunnel: [w784 w792] -> _
              tunnel: w774 -> [_ w796]
              tunnel: w773 -> [_ w795]
              tunnel: [w783 w791] -> w772
              frame False {
                n118 = call "DB insert array data（Feedback).vi"("Data"=w786, "error in (no error)"=w790, "index"=0, "table"=w788, "Connncet State"=w789) -> ("error out"=w785:errorcluster, "state"=w783:bool, "Connncet State out"=w784:T6)  [unwired: 4 in]
              }
              frame True {
                n119 = call "DB Update Data(Feedback).vi"("Pos"=cluster{"index":i32, "Len":i32} {"index"=0, "Len"=14}, "Sel index"=0, "data"=w795, "error in (no error)"=w799, "Code"=w796, "table"=w797, "Connncet State"=w798) -> ("error out"=w793:errorcluster, "State"=w791:bool, "Connncet State out"=w792:T6)  [unwired: 2 in]
              }
            }
          }
        }
        n120 = call "Error cyc Times.vi"("error in (no error)"=w755, "Status in"=w754) -> ("error out"=w743:errorcluster, "Numeric"=w749:i32, "Cys Status"=w752:bool, "Status out"=w734:bool)  [unwired: 6 in]
        n121 = Equal?(x=w749, y=2) -> (x = y?=w747:bool)
        n122 = Select(t="尾站_SN:%2$s的FTT_Write表数据记录异常！", s=w734, f="尾站_SN:%2$sNG数据记录完成！") -> (s? t:f=w733:string)
        n123 = Format Into String(format string=w733, error in=w743, w742, w740) -> (resulting string=w738:string, error out=w739:errorcluster)  [unwired: 1 in]
        n124 = Bundle By Name(cluster=w745, "information.cause"=w738, "Display"=T9 {"Line.No"="", "Model"="", "Color"="", "UPH"=0.0, "Plan"=0.0, "Target Rate"=0.0, "Target "=0.0, "Actual"=0.0, "FTT"=0.0, "FTT Rate"=0.0, "Repaired"=0.0, "Reject"=0.0, "Ouline"=0.0, "Line State"=""}) -> (w744:T12)
        n125 = Select(t=string[] ["FTT:Data Save", "Display Tip"], s=w747, f=string[] ["FTT:Data Save"]) -> (s? t:f=w750:string[])
        n126 = Not(x=w752) -> (.not. x?=w753:bool)
      }
      frame "FTT:Close database" {
        n127 = Unbundle By Name(w802) -> ("Main.Local DB.Database"=w804:T6)
        n128 = call "Disconncetion DB.vi"("error in (no error)"=w806, "Connncet State"=w804) -> ("error out"=w805:errorcluster, "Connect State"=w803:T6)  [unwired: 8 in]
        n129 = Bundle By Name(cluster=w802, "Main.Local DB.Database"=w803) -> (w801:T12)
      }
      frame "Scan:Scank Feedback" {
        n130 = call "Write Sigle Bool.vi"("error in (no error)"=w811, "Data"=TRUE, "Tags"="Write_Sign") -> ("error out"=w810:errorcluster)  [unwired: 6 in, 2 out]
      }
      frame "Complete Steps" {
      }
      frame "Quit" {
      }
      frame "Input & Ouput" {
        n131 = Unbundle By Name(w828) -> ("Main.Ctr.Exit"=w826:refnum<vi>)
        n132 = property class="Bool (严格)"(reference=w826, error in=w827) -> (error out=w825:errorcluster, "Value"=w823:bool)  [unwired: 1 out]
      }
      frame "Display Tip" {
        n133 = Unbundle By Name(w837) -> ("information"=w831:T10)
        n134 = Unbundle By Name(w832) -> ("source"=w830:string)
        n135 = Bundle By Name(cluster=w831, "Suroce"=w830) -> (w829:T10)
        n136 = call "Log info.vi"("error in (no error)"=w832, "information"=w829) -> ("error out"=w834:errorcluster)  [unwired: 8 in, 1 out]
        n137 = call <vilib>:"Clear Errors.vi"("error in (no error)"=w834) -> ("error out"=w833:errorcluster)  [unwired: 5 in, 1 out]
      }
      frame "Error Log" {
        n138 = Unbundle By Name(w847) -> ("information"=w846:T10)
        n139 = Unbundle By Name(w842) -> ("source"=w840:string, "code"=w841:i32)
        n140 = Bundle By Name(cluster=w846, "Status"=TRUE, "Suroce"=w840, "code"=w841) -> (w845:T10)
        n141 = call "Log info.vi"("error in (no error)"=w842, "information"=w845) -> ("error out"=w849:errorcluster)  [unwired: 8 in, 1 out]
        n142 = call <vilib>:"Clear Errors.vi"("error in (no error)"=w849) -> ("error out"=w848:errorcluster)  [unwired: 5 in, 1 out]
      }
    }
    n143 = call "Insert Multiple Events(Error).vi"("error in (no error)"=w12, "Insert all? (T)"=w15, "Events to Insert"=w14, "Event queue in"=w16) -> ("error out"=w11:errorcluster, "Event queue out"=w17:string[])  [unwired: 6 in]
  }
  "error out" <- w3
